vi "Set Boolean.vi"(7 "Name":string="Set Boolean", 10 "Boolean Value":bool, 11 "Abs_Boolean.lvclass":refnum<class "Abs_Boolean.lvclass">) -> (3 "Node":refnum<class "abs_Node.lvclass">)   [LabVIEW 2021, in "BT.lvlib"]
uses:
  BT.lvlib
  Support/abs_Node/abs_Node.lvclass
  LV_Abstract/Source/Abs_Types/Boolean/Abs_Boolean.lvclass
  C:/Users/Tim/Documents/GitHub/LV_Abstract/Source/Abs_Types/Type/Abs_Type.lvclass
  Support/Set Boolean/Set Boolean.lvclass
  C:/Users/Tim/Documents/GitHub/LV_Behaviour_Tree/Source/Support/abs_Type Leaf/abs_Type Leaf.lvclass
  C:/Users/Tim/Documents/GitHub/LV_Behaviour_Tree/Source/Support/abs_Node/abs_Node.lvclass
  Support/abs_Type Leaf/abs_Type Leaf.lvclass/abs_Type Leaf.ctl
  LV_Abstract/Source/Abs_Types/Type/Abs_Type.lvclass/Abs_Type.ctl
  Support/Set Boolean/Set Boolean.lvclass/Set Boolean.ctl
  Support/abs_Type Leaf/Properties/Write Value Class.vi
  LV_Abstract/Source/Abs_Types/Type/Properties/Write Name.vi
  Support/Set Boolean/Properties/Write Boolean.vi
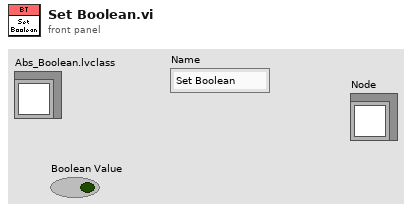
[diagram p1: front panel]
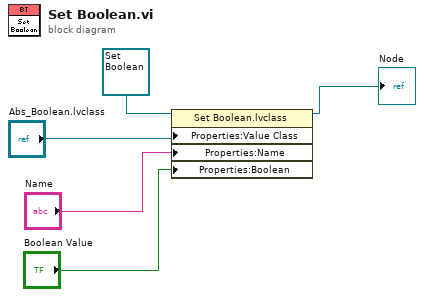
[diagram p0: block diagram]
diagram:
  n1 = property class="Set Boolean.lvclass"(reference=refnum<class "Set Boolean.lvclass"> refnum ("BT.lvlib:Set Boolean.lvclass"), "Properties:Value Class"="Abs_Boolean.lvclass", "Properties:Name"="Name", "Properties:Boolean"="Boolean Value") -> (reference out=→"Node":refnum<class "Set Boolean.lvclass">)  [unwired: 1 in, 1 out]
